vi "Search by SN.vi"(10 "Device Info":T1, 11 "array of devices":T2) -> (3 "index of element":i32)   [LabVIEW 2016]
uses:
  Array Device Info.ctl
  Device Info.ctl
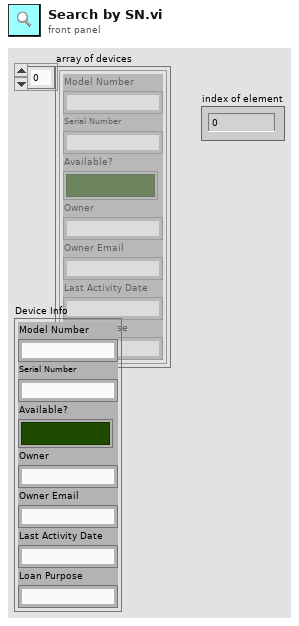
[diagram p1: front panel]
types:
  T1 = typedef "Device Info.ctl" = cluster{"Model Number":string, "Serial Number":string, "Available?":bool, "Owner":string, "Owner Email":string, "Last Activity Date":string, "Loan Purpose":string}
  T2 = typedef "Array Device Info.ctl" = T1[]
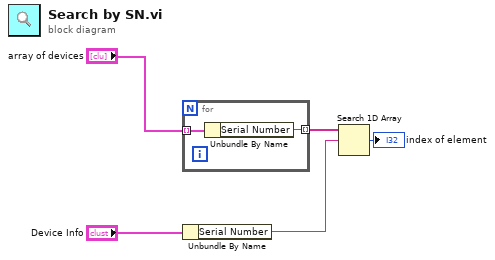
[diagram p0: block diagram]
diagram:
  n1 = for {
    tunnel: "array of devices" -> [w7] mode=indexing
    tunnel: [w6] -> w2 mode=indexing
    n2 = Unbundle By Name(w7) -> ("Serial Number"=w6:string)
  }
  n3 = Unbundle By Name("Device Info") -> ("Serial Number"=w3:string)
  n4 = Search 1D Array(1D array=w2, element=w3) -> (index of element=→"index of element":i32)  [unwired: 1 in]
